vi "Salaire.vi"(3 "Taux horaire":dbl, 4 "Tableau heures fin employé":timestamp[](array[timestamp]), 5 "Tableau heures debut employé":timestamp[](array[timestamp]), 6 "button calc salaire":bool) -> (0 "Cout des salaires":dbl, 1 "Salaire net":dbl, 2 "Salaire brut":dbl)   [LabVIEW 2024]
uses:
  <vilib>/express/express shared/transition.llb/Dynamic To Waveform Array.vi
  <vilib>/express/express signal manip/GetorSetDDTAttributes/Set DDT Attributes/SetT0.vi
  <vilib>/express/express shared/transition.llb/Waveform Array To Dynamic.vi
  charge_salairial.vi
  <vilib>/express/express signal manip/GetorSetDDTAttributes/Set DDT Attributes/Set DDT Properties.xnode
panel:
  out "check charge salairial":dbl
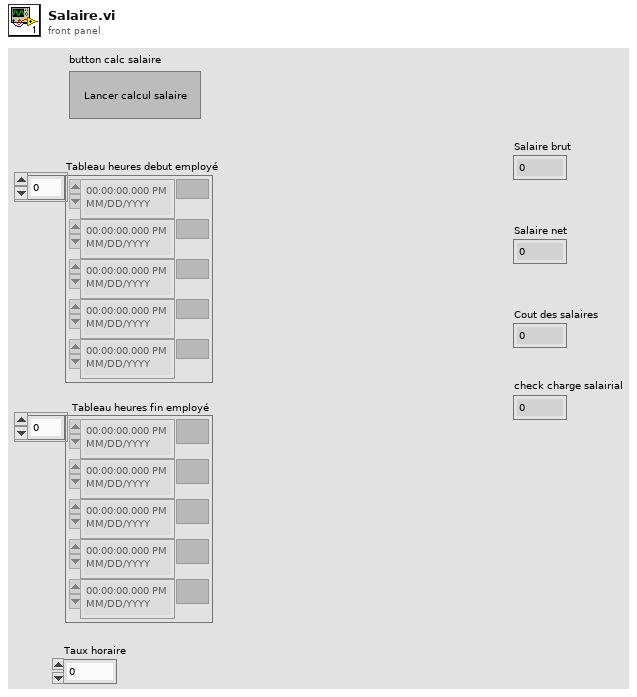
[diagram p1: front panel]
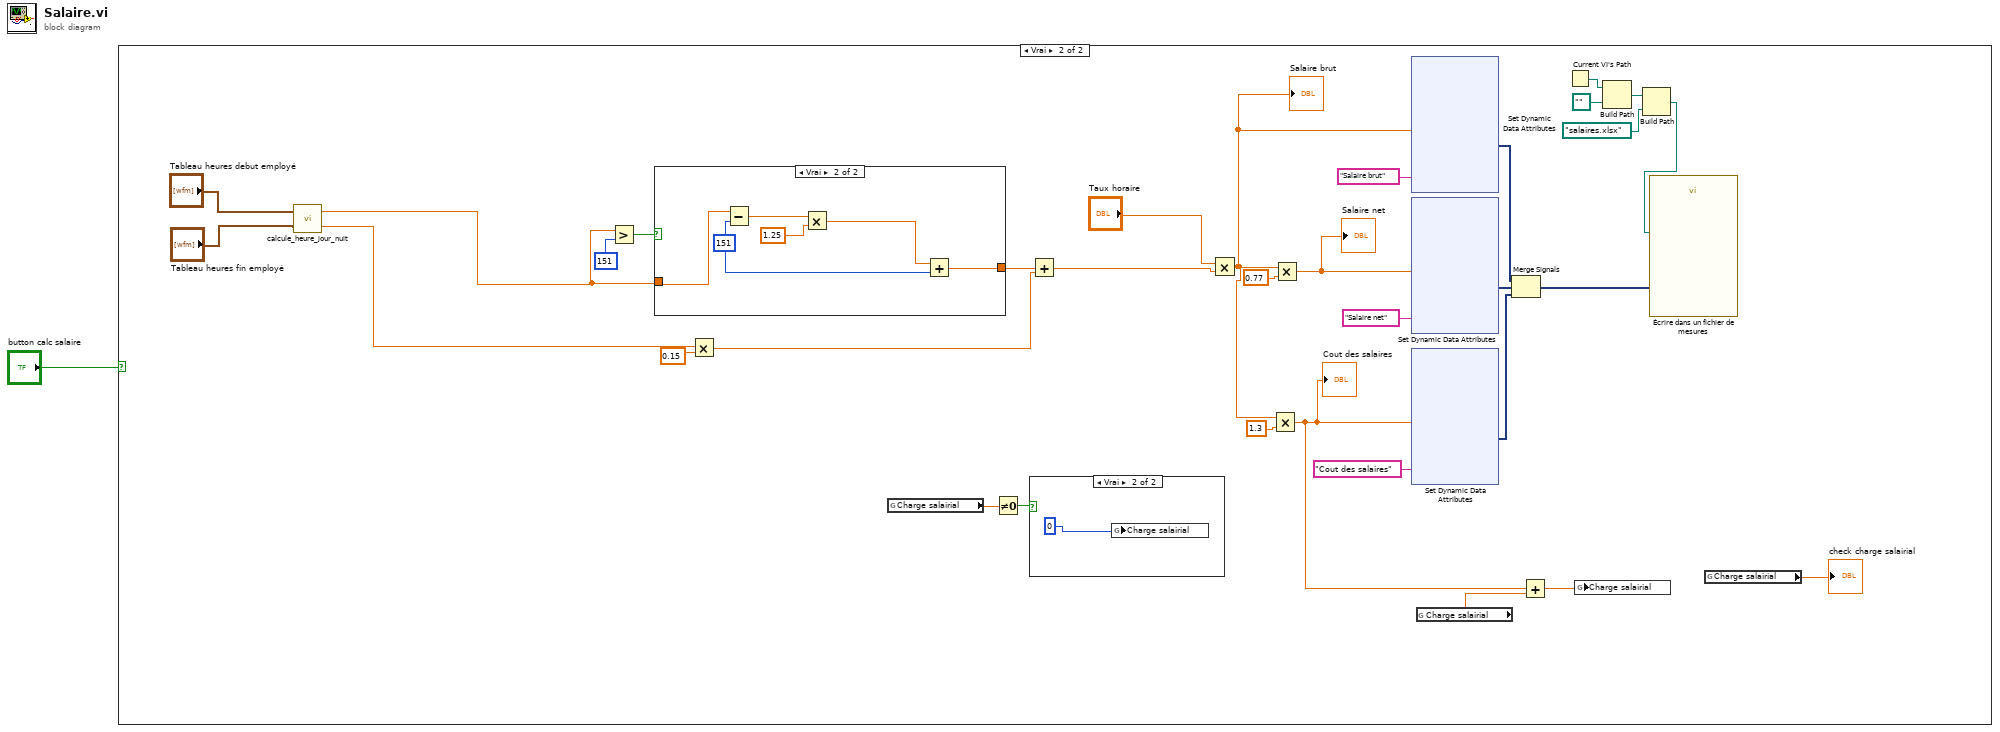
[diagram p0: block diagram]
diagram:
  n1 = case shown="Vrai" "button calc salaire" {
    frame False {
    }
    frame True {
      n2 = call "calcule_heure_jour_nuit.vi"("Tableau fin"="Tableau heures fin employé", "Tableau debut"="Tableau heures debut employé") -> ("nombre heures nuit"=w14:dbl, "nombre heures jour"=w15:dbl)
      n3 = Greater?(x=w15, y=151) -> (0:w20:bool)
      n4 = case shown="Vrai" w20 {
        tunnel: w15 -> [w35 w37]
        tunnel: [w35 w38] -> w17
        frame False {
        }
        frame True {
          w36 = 151
          n5 = Subtract(x=w37, y=w36) -> (x-y=w41:dbl)
          n6 = Multiply(x=w41, y=1.25) -> (x*y=w39:dbl)
          n7 = Add(x=w39, y=w36) -> (x+y=w38:dbl)
        }
      }
      n8 = Multiply(x=w14, y=0.15) -> (x*y=w16:dbl)
      n9 = global read "charge_salairial.vi" "Charge salairial"() -> (w24:dbl)
      n10 = Not Equal To 0?(x=w24) -> (x != 0?=w23:bool)
      n11 = Add(x=w17, y=w16) -> (x+y=w12:dbl)
      n12 = case shown="Vrai" w23 {
        frame False {
        }
        frame True {
          n13 = global write "charge_salairial.vi" "Charge salairial"(0) -> ()
        }
      }
      n14 = Multiply(x="Taux horaire", y=w12) -> (x*y=w11:dbl)
      "Salaire brut" <- w11
      n15 = Multiply(x=w11, y=1.3) -> (x*y=w7:dbl)
      "Cout des salaires" <- w7
      n16 = Multiply(x=w11, y=0.77) -> (x*y=w10:dbl)
      "Salaire net" <- w10
      n17 = xnode "Set Dynamic Data Attributes"("Signals In"=w11, "Signal Name"="Salaire brut" ("String")) -> ("Signals Out"=w30:dynamicdata)  [unwired: 2 in, 1 out]
      n18 = xnode "Set Dynamic Data Attributes"("Signals In"=w10, "Signal Name"="Salaire net" ("String")) -> ("Signals Out"=w27:dynamicdata)  [unwired: 2 in, 1 out]
      n19 = xnode "Set Dynamic Data Attributes"("Signals In"=w7, "Signal Name"="Cout des salaires" ("String")) -> ("Signals Out"=w26:dynamicdata)  [unwired: 2 in, 1 out]
      n20 = global read "charge_salairial.vi" "Charge salairial"() -> (w9:dbl)
      n21 = Merge Signals(w30, w27, w26) -> (w32:dynamicdata)
      n22 = Add(x=w7, y=w9) -> (x+y=w8:dbl)
      n23 = Current VI's Path() -> (path=w6:path)
      n24 = global write "charge_salairial.vi" "Charge salairial"(w8) -> ()
      n25 = Build Path(base path=w6, name or relative path=path "..") -> (appended path=w3:path)
      n26 = Build Path(base path=w3, name or relative path=path "salaires.xlsx" ("Filename")) -> (appended path=w2:path)
      n27 = call "Écrire dans un fichier de mesures"("Signals"=w32, "Filename"=w2) -> ()  [unwired: 15 in, 3 out]
      n28 = global read "charge_salairial.vi" "Charge salairial"() -> (→"check charge salairial":dbl)
    }
  }
